vi "HermitePolynomial.vi"(1 "n":i16, 2 "x":dbl format="%.2f") -> (0 "Hermite polynomial (n,x)":dbl format="%.2f")   [LabVIEW 2024]
uses:
  <vilib>/gmath/NI_Gmath.lvlib
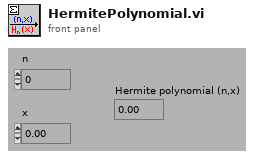
[diagram p1: front panel]
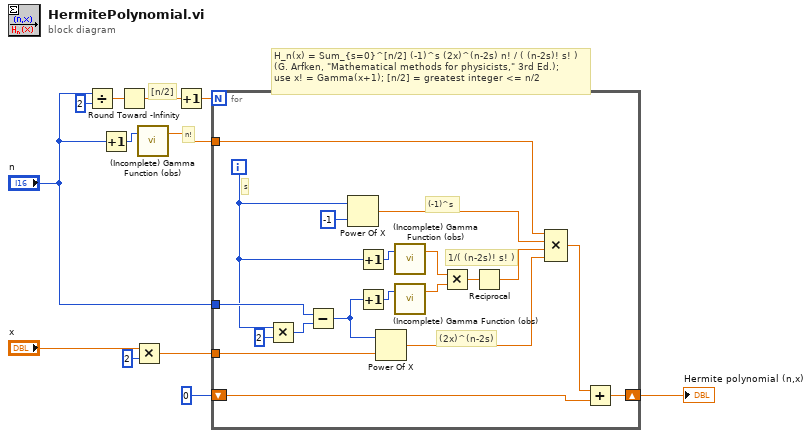
[diagram p0: block diagram]
diagram:
  # "n!"
  # "[n/2]"
  # "H_n(x) = Sum_{s=0}^[n/2] (-1)^s (2x)^(n-2s) n! / ( (n-2s)! s! )\n(G. Arfken, \"Mathematical methods for physicists,\" 3rd Ed.);\nuse x! = Gamma(x+1); [n/2] = greatest integer <= n/2"
  n1 = Divide(x="n", y=2) -> (x/y=w6:dbl)
  n2 = Increment(x="n") -> (x+1=w1:i16)
  n3 = Round Toward -Infinity(1:w6) -> (0:w7:dbl)
  n4 = Multiply(x="x", y=2) -> (x*y=w4:dbl)
  n5 = call <vilib>:"(Incomplete) Gamma Function (obs).vi"("x"=w1) -> ("g(x, a)"=w11:dbl)  [unwired: 2 in]
  n6 = Increment(x=w7) -> (x+1=w12:dbl)
  n7 = for {
    N: w12 -> [_]
    tunnel: "n" -> [w26]
    tunnel: w11 -> [w17]
    tunnel: w4 -> [w31]
    shift-right: [w30] -> w9
    shift-left: 0 -> [w29]
    i -> [w21]
    # "1/( (n-2s)! s! )"
    # "(2x)^(n-2s)"
    # "(-1)^s"
    # "s"
    n8 = Multiply(x=w21, y=2) -> (x*y=w27:i32)
    n9 = Subtract(x=w26, y=w27) -> (x-y=w25:i32)
    n10 = Power Of X(1:-1, 2:w21) -> (0:w19:dbl)
    n11 = Increment(x=w21) -> (x+1=w14:i32)
    n12 = Increment(x=w25) -> (x+1=w13:i32)
    n13 = Power Of X(1:w31, 2:w25) -> (0:w18:dbl)
    n14 = call <vilib>:"(Incomplete) Gamma Function (obs).vi"("x"=w14) -> ("g(x, a)"=w24:dbl)  [unwired: 2 in]
    n15 = call <vilib>:"(Incomplete) Gamma Function (obs).vi"("x"=w13) -> ("g(x, a)"=w23:dbl)  [unwired: 2 in]
    n16 = Multiply(x=w24, y=w23) -> (x*y=w20:dbl)
    n17 = Reciprocal(x=w20) -> (1/x=w16:dbl)
    n18 = Compound Arithmetic op=MULTIPLY(w17, w19, w16, w18) -> (w15:dbl)
    n19 = Add(x=w15, y=w29) -> (x+y=w30:dbl)
  }
  "Hermite polynomial (n,x)" <- w9
